vi "PID.vi"(0 "process variable":dbl format="%.2f", 1 "setpoint":dbl format="%.2f", 2 "PID gains":T1={"proportional gain (Kc)"=1.0, "integral time (Ti, min)"=0.01, "derivative time (Td, min)"=0.0} {"derivative time (Td, min)" format="%.3f"; "integral time (Ti, min)" format="%.3f"; "proportional gain (Kc)" format="%.3f"}, 3 "dt (s)":dbl=-1.0 format="%.3f", 4 "reinitialize? (F)":bool) -> (5 "LeftPower":dbl, 6 "RightPower":dbl, 7 "Done":bool)   [LabVIEW 2016]
uses:
  <vilib>/addons/control/pid/pid.llb/PID (DBL).vi
  <vilib>/Rock Robotics/Network Tables/NT Write Number.vi
  <vilib>/addons/control/pid/NI_PID_pid.lvlib
panel:
  out "coerced(x)":dbl
  in  "ErrorRange":dbl=0.5
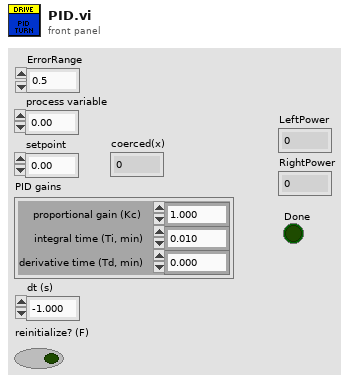
[diagram p1: front panel]
types:
  T1 = cluster{"proportional gain (Kc)":dbl, "integral time (Ti, min)":dbl, "derivative time (Td, min)":dbl}
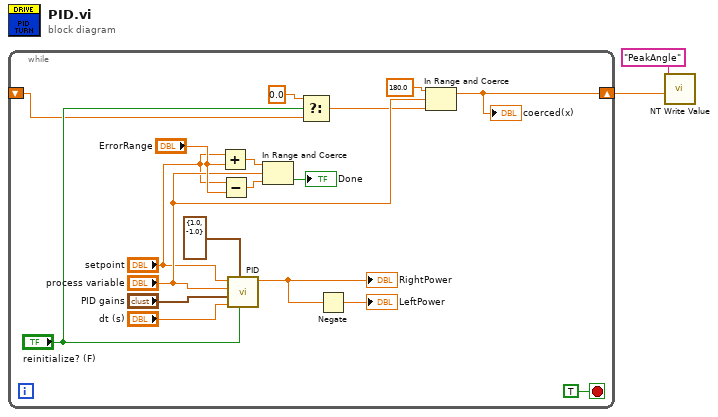
[diagram p0: block diagram]
diagram:
  n1 = while {
    shift-right: [w11] -> w2
    shift-left: _ -> [w8]
    stop <- TRUE stop-if-true
    n2 = Add(x="setpoint", y="ErrorRange") -> (x+y=w17:dbl)
    n3 = Subtract(x="setpoint", y="ErrorRange") -> (x-y=w16:dbl)
    n4 = call-poly <vilib>:"PID.vi"("reinitialize? (F)"="reinitialize? (F)", "output range"=cluster{"output high":dbl, "output low":dbl} {"output high"=1.0, "output low"=-1.0}, "dt (s)"="dt (s)", "PID gains"="PID gains", "process variable"="process variable", "setpoint"="setpoint") -> ("output"=w4:dbl)  [unwired: 4 in, 1 out]
    "RightPower" <- w4
    n5 = In Range and Coerce(upper limit=w17, x="process variable", lower limit=w16) -> (In Range?=→"Done":bool)  [unwired: 1 out]
    n6 = Select(t=0.0, s="reinitialize? (F)", f=w8) -> (s? t:f=w7:dbl)
    n7 = Negate(x=w4) -> (-x=→"LeftPower":dbl)
    n8 = In Range and Coerce(upper limit=180.0, x="process variable", lower limit=w7) -> (coerced(x)=w11:dbl)  [unwired: 1 out]
    "coerced(x)" <- w11
  }
  n9 = call-poly <vilib>:"NT Write Value.vi"("Numeric"=w2, "Name"="PeakAngle") -> ()  [unwired: 9 in, 1 out]
